vi "SetupUserMem.vi"(2 "blocks":u32=1, 3 "nos":u32=1, 4 "Board_sel":u32=1) -> ()   [LabVIEW 2015]
uses:
  ESLSCDLL.dll
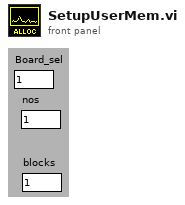
[diagram p1: front panel]
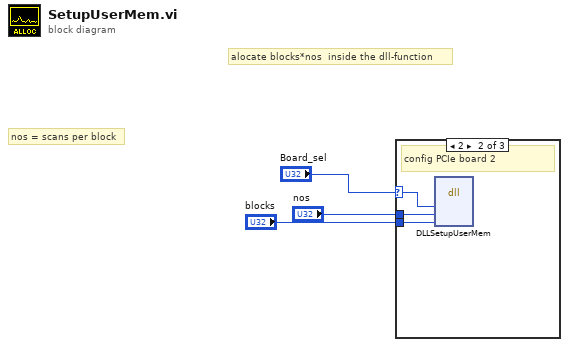
[diagram p0: block diagram]
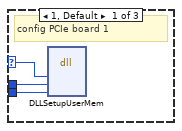
[diagram p2: hidden frame]
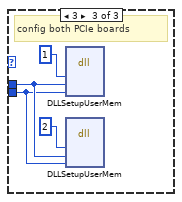
[diagram p3: hidden frame]
diagram:
  # "alocate blocks*nos  inside the dll-function"
  # "nos = scans per block"
  n1 = case shown="2" "Board_sel" {
    selector: "Board_sel" -> [w6 w7 _]
    tunnel: "blocks" -> [w5 w9 w10]
    tunnel: "nos" -> [w4 w8 w11]
    frame 1, Default {
      # "config PCIe board 1"
      n2 = dll-call lib="C:/Users/Gerhard/ENTW/PCIE/64bit/lv64/board.vis/ESLSCDLL.dll" fn="DLLSetupUserMem" ("lwlscdll.dll:DLLReadFFLoop")("drv"=w6, "nos"=w4, "nob"=w5) -> ()  [unwired: 7 in, 2 out]
    }
    frame 2 {
      # "config PCIe board 2"
      n3 = dll-call lib="C:/Users/Gerhard/ENTW/PCIE/64bit/lv64/board.vis/ESLSCDLL.dll" fn="DLLSetupUserMem" ("lwlscdll.dll:DLLReadFFLoop")("drv"=w7, "nos"=w8, "nob"=w9) -> ()  [unwired: 7 in, 2 out]
    }
    frame 3 {
      # "config both PCIe boards"
      n4 = dll-call lib="C:/Users/Gerhard/ENTW/PCIE/64bit/lv64/board.vis/ESLSCDLL.dll" fn="DLLSetupUserMem" ("lwlscdll.dll:DLLReadFFLoop")("drv"=u32 1, "nos"=w11, "nob"=w10) -> ()  [unwired: 7 in, 2 out]
      n5 = dll-call lib="C:/Users/Gerhard/ENTW/PCIE/64bit/lv64/board.vis/ESLSCDLL.dll" fn="DLLSetupUserMem" ("lwlscdll.dll:DLLReadFFLoop")("drv"=u32 2, "nos"=w11, "nob"=w10) -> ()  [unwired: 7 in, 2 out]
    }
  }
